vi "00 DoubleCheck.vi"(8 "error in (no error)":errorcluster caption="错误输入（无错误）", 10 "客服端参数":cluster{"本机端口":u16, "主机 IP":string, "主机端口":u16}={"本机端口"=0, "主机 IP"="0", "主机端口"=0}, 11 "TCPClientClass 输入":refnum<class "TCPClientClass.lvclass">) -> (0 "error out":errorcluster caption="错误输出", 1 "端口重复？":bool, 2 "参数重复？":bool, 3 "TCPClientClass 输出":refnum<class "TCPClientClass.lvclass">)   [LabVIEW 2019, in "TCPClientClass.lvclass"]
uses:
  TCPClientClass.lvclass
  TCPClientClass.lvclass/TCPClientClass.ctl
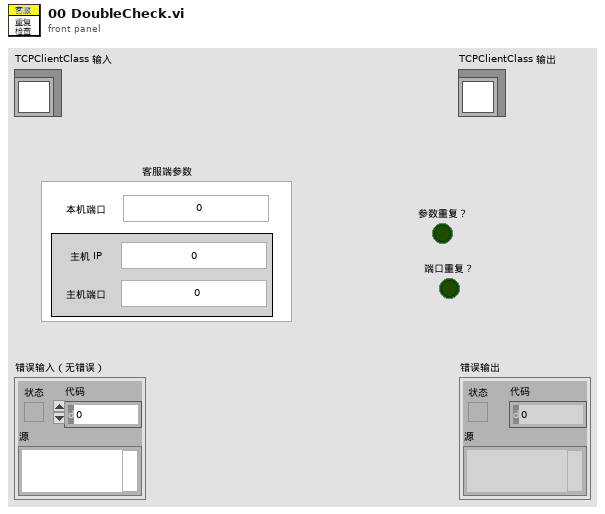
[diagram p1: front panel]
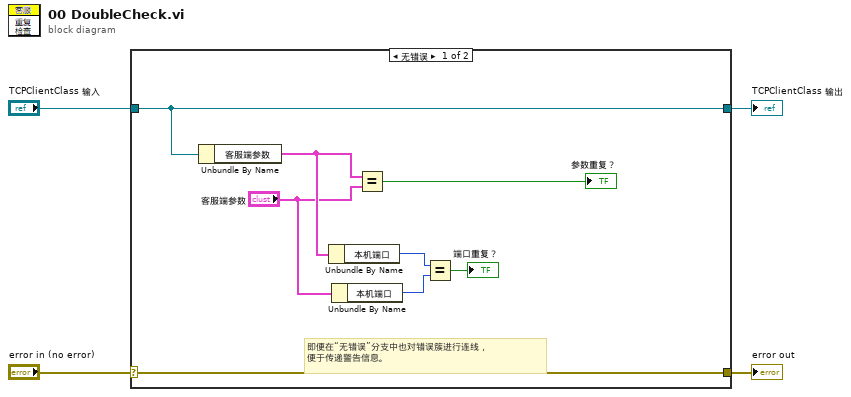
[diagram p0: block diagram]
diagram:
  n1 = case shown="无错误" "error in (no error)" {
    selector: "error in (no error)" -> [w12 w14]
    tunnel: [w12 w14] -> w3
    tunnel: [w11 w13] -> w1
    tunnel: "TCPClientClass 输入" -> [w11 w13]
    frame No Error {
      # "即便在“无错误”分支中也对错误簇进行连线，\n便于传递警告信息。"
      n2 = Unbundle By Name(w11) -> ("客服端参数"=w9:cluster{"本机端口":u16, "主机 IP":string, "主机端口":u16})
      n3 = Unbundle By Name(w9) -> ("本机端口"=w7:u16)
      n4 = Unbundle By Name("客服端参数") -> ("本机端口"=w6:u16)
      n5 = Equal?(x=w9, y="客服端参数") -> (x = y?=→"参数重复？":bool)
      n6 = Equal?(x=w7, y=w6) -> (x = y?=→"端口重复？":bool)
    }
    frame Error {
    }
  }
  "error out" <- w3
  "TCPClientClass 输出" <- w1
